vi "navX x_y_z (SubVI).vi"(0 "I2C Ref Out in":T1, 11 "error in (no error)":errorcluster) -> (4 "I2C Ref Out out":T1, 6 "value Z":ext, 8 "value Y":ext, 10 "value X":ext, 15 "error out":errorcluster)   [LabVIEW 2017]
uses:
  <vilib>/myRIO/Instrument Drivers/Onboard IO/I2C/typedefs/I2C Reference.ctl
  <vilib>/myRIO/Common/Instrument Driver Framework/Utilities/typedefs/myRIO Generic Hardware Reference.ctl
  <vilib>/myRIO/Common/Instrument Driver Framework/Utilities/typedefs/Hardware Version Enum.ctl
  <vilib>/myRIO/Common/Instrument Driver Framework/Utilities/typedefs/myRIO v1.0 Reference.ctl
  <vilib>/myRIO/Common/Instrument Driver Framework/Utilities/typedefs/Generic FPGA Reference.ctl
  <vilib>/myRIO/Common/Instrument Driver Framework/myRIO v1.0/I2C/typedefs/I2C Channels Enum.ctl
  <vilib>/myRIO/Instrument Drivers/Onboard IO/I2C/typedefs/I2C Configuration.ctl
  <vilib>/myRIO/Instrument Drivers/Onboard IO/I2C/typedefs/I2C Transfer Rate.ctl
  <vilib>/Utility/error.llb/Error Cluster From Error Code.vi
  <vilib>/myRIO/Common/Instrument Driver Framework/myRIO v1.0/I2C/vis/myRIO v1.0 Write I2C.vi
  <vilib>/myRIO/Common/Instrument Driver Framework/myRIO v1.0/I2C/vis/myRIO v1.0 Read I2C.vi
  <vilib>/myRIO/Instrument Drivers/Onboard IO/I2C/I2C.lvlib
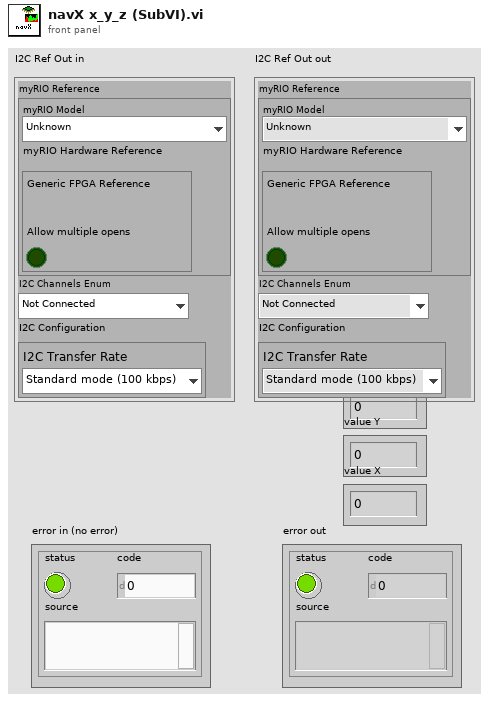
[diagram p1: front panel]
types:
  T1 = typedef "I2C.lvlib/I2C Reference.ctl" = cluster{"myRIO Reference":T2, "I2C Channels Enum":T6, "I2C Configuration":T7}
  T2 = typedef "myRIO Generic Hardware Reference.ctl" = cluster{"myRIO Model":T3, "myRIO Hardware Reference":T4}
  T3 = typedef "Hardware Version Enum.ctl" = enum16{"Unknown", "myRIO-1900", "myRIO-1950", "roboRIO", "NI ELVIS RIO CM"}
  T4 = typedef "myRIO v1.0 Reference.ctl" = cluster{"Generic FPGA Reference":T5, "Allow multiple opens":bool}
  T5 = typedef "Generic FPGA Reference.ctl" = refnum<k20>
  T6 = typedef "I2C Channels Enum.ctl" = enum16{"Not Connected", "A/I2C", "B/I2C", "I2C/I2C"}
  T7 = typedef "I2C.lvlib/I2C Configuration.ctl" = cluster{"I2C Transfer Rate":T8}
  T8 = typedef "I2C.lvlib/I2C Transfer Rate.ctl" = enum16{"Standard mode (100 kbps)", "Fast mode (400 kbps)"}
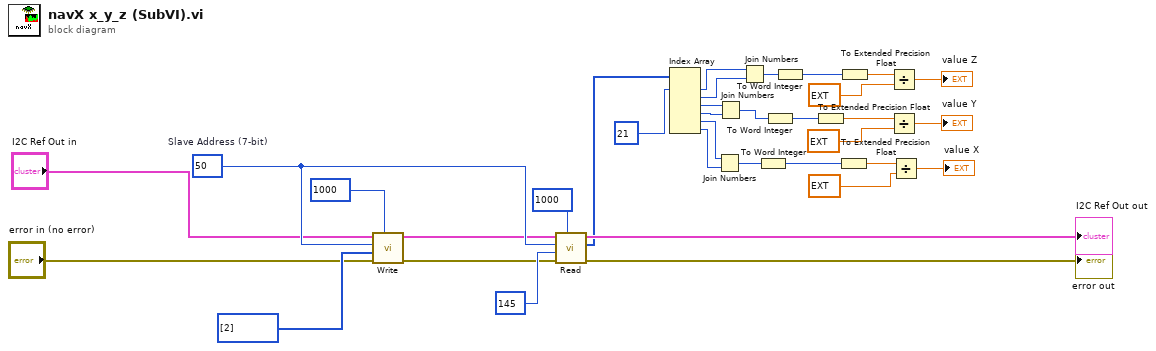
[diagram p0: block diagram]
diagram:
  w9 = u8 50  # Slave Address (7-bit)
  n1 = call <vilib>:"Write.vi"("Timeout ms (1000)"=1000, "error in (no error)"="error in (no error)", "Bytes to Write"=u8[] [2], "Slave Address (7-bit)"=w9, "I2C Ref In"="I2C Ref Out in") -> ("error out"=w3:errorcluster, "I2C Ref Out"=w5:T1)  [unwired: 5 in]
  n2 = call <vilib>:"Read.vi"("Timeout ms (1000)"=1000, "error in (no error)"=w3, "Byte Count"=u32 145, "Slave Address (7-bit)"=w9, "I2C Ref In"=w5) -> ("error out"=→"error out":errorcluster, "Bytes Read"=w10:u8[], "I2C Ref Out"=→"I2C Ref Out out":T1)  [unwired: 3 in]
  n3 = Index Array(array=w10, index #1=21 ("index")) -> (element #1=w15:u8, element #2=w12:u8, element #3=w17:u8, element #4=w18:u8, element #5=w20:u8, element #6=w21:u8)  [unwired: 5 in]
  n4 = Join Numbers(hi=w20, lo=w21) -> ((hi.lo)=w19:u16)
  n5 = Join Numbers(hi=w17, lo=w18) -> ((hi.lo)=w16:u16)
  n6 = Join Numbers(hi=w15, lo=w12) -> ((hi.lo)=w11:u16)
  n7 = To Word Integer(number=w19) -> (16bit integer=w23:i16)
  n8 = To Word Integer(number=w16) -> (16bit integer=w22:i16)
  n9 = To Word Integer(number=w11) -> (16bit integer=w13:i16)
  n10 = To Extended Precision Float(1:w22) -> (0:w27:ext)
  n11 = To Extended Precision Float(1:w23) -> (0:w29:ext)
  n12 = To Extended Precision Float(1:w13) -> (0:w28:ext)
  n13 = Divide(x=w28, y=ext 100.0) -> (x/y=→"value Z":ext)
  n14 = Divide(x=w27, y=ext 100.0) -> (x/y=→"value Y":ext)
  n15 = Divide(x=w29, y=ext 100.0) -> (x/y=→"value X":ext)
